vi "QueryLimitTripOffLCDC501.vi"(8 "error in (no error)":errorcluster, 11 "VISA resource name":refnum<visa-resource-name>) -> (0 "error out":errorcluster, 2 "LASER LIMIT & TRIP-OFF":T1, 3 "VISA resource name out":refnum<visa-resource-name>)   [LabVIEW 2021]
panel:
  # "Laser Trip-off on"
  # "Current Limit"
  # "TEC Off"
  # "Min Temperature"
  # "Max Temperature"
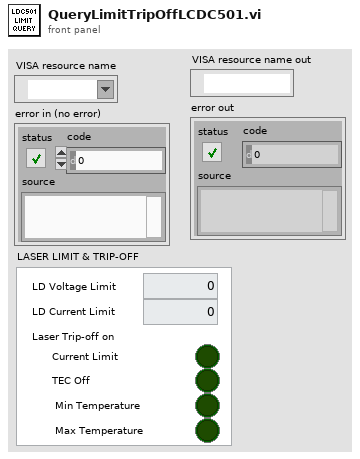
[diagram p1: front panel]
types:
  T1 = cluster{"LD Voltage Limit":dbl, "LD Current Limit":dbl, "Laser Trip-off on Current Limit":bool, "Laser Trip-off on TEC Off":bool, "Laser Trip-off on Min Temperature":bool, "Laser Trip-off on Max Temperature":bool}
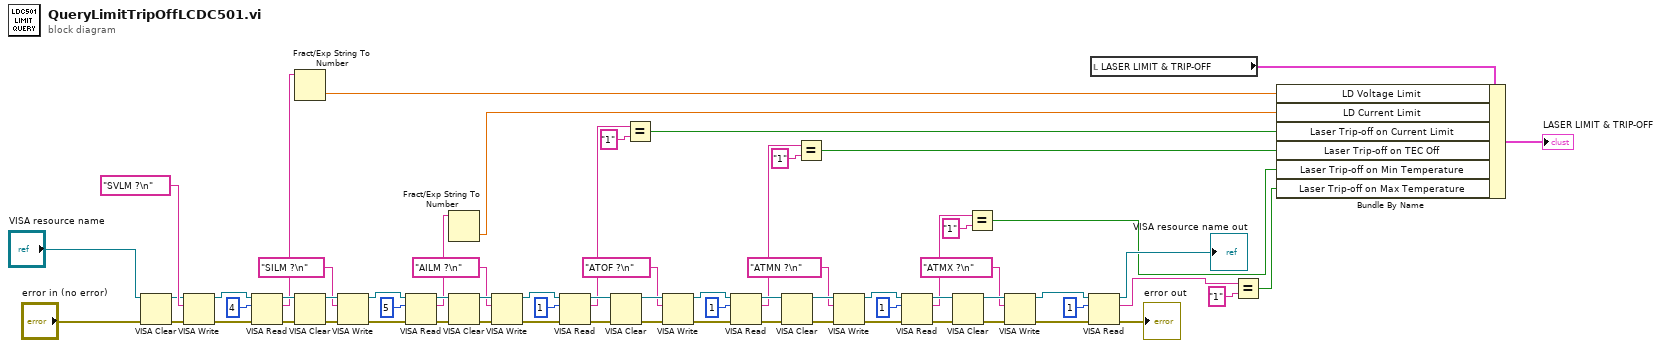
[diagram p0: block diagram]
diagram:
  n1 = VISA Clear(VISA resource name="VISA resource name", error in (no error)="error in (no error)") -> (VISA resource name out=w63:refnum<visa-resource-name>, error out=w64:errorcluster)
  n2 = VISA Write(VISA resource name=w63, write buffer="SVLM ?\n", error in (no error)=w64) -> (VISA resource name out=w67:refnum<visa-resource-name>, error out=w66:errorcluster)  [unwired: 1 out]
  n3 = VISA Read(VISA resource name=w67, byte count=u32 4, error in (no error)=w66) -> (VISA resource name out=w40:refnum<visa-resource-name>, read buffer=w18:string, error out=w39:errorcluster)  [unwired: 1 out]
  n4 = Fract/Exp String To Number(string=w18) -> (number=w8:dbl)  [unwired: 3 in, 1 out]
  n5 = VISA Clear(VISA resource name=w40, error in (no error)=w39) -> (VISA resource name out=w59:refnum<visa-resource-name>, error out=w60:errorcluster)
  n6 = VISA Write(VISA resource name=w59, write buffer="SILM ?\n", error in (no error)=w60) -> (VISA resource name out=w62:refnum<visa-resource-name>, error out=w61:errorcluster)  [unwired: 1 out]
  n7 = VISA Read(VISA resource name=w62, byte count=u32 5, error in (no error)=w61) -> (VISA resource name out=w55:refnum<visa-resource-name>, read buffer=w17:string, error out=w53:errorcluster)  [unwired: 1 out]
  n8 = Fract/Exp String To Number(string=w17) -> (number=w6:dbl)  [unwired: 3 in, 1 out]
  n9 = VISA Clear(VISA resource name=w55, error in (no error)=w53) -> (VISA resource name out=w54:refnum<visa-resource-name>, error out=w56:errorcluster)
  n10 = VISA Write(VISA resource name=w54, write buffer="AILM ?\n", error in (no error)=w56) -> (VISA resource name out=w57:refnum<visa-resource-name>, error out=w58:errorcluster)  [unwired: 1 out]
  n11 = VISA Read(VISA resource name=w57, byte count=u32 1, error in (no error)=w58) -> (VISA resource name out=w48:refnum<visa-resource-name>, read buffer=w15:string, error out=w47:errorcluster)  [unwired: 1 out]
  n12 = VISA Clear(VISA resource name=w48, error in (no error)=w47) -> (VISA resource name out=w49:refnum<visa-resource-name>, error out=w50:errorcluster)
  n13 = Equal?(x=w15, y="1") -> (x = y?=w5:bool)
  n14 = VISA Write(VISA resource name=w49, write buffer="ATOF ?\n", error in (no error)=w50) -> (VISA resource name out=w51:refnum<visa-resource-name>, error out=w52:errorcluster)  [unwired: 1 out]
  n15 = VISA Read(VISA resource name=w51, byte count=u32 1, error in (no error)=w52) -> (VISA resource name out=w44:refnum<visa-resource-name>, read buffer=w13:string, error out=w41:errorcluster)  [unwired: 1 out]
  n16 = VISA Clear(VISA resource name=w44, error in (no error)=w41) -> (VISA resource name out=w43:refnum<visa-resource-name>, error out=w45:errorcluster)
  n17 = Equal?(x=w13, y="1") -> (x = y?=w4:bool)
  n18 = VISA Write(VISA resource name=w43, write buffer="ATMN ?\n", error in (no error)=w45) -> (VISA resource name out=w42:refnum<visa-resource-name>, error out=w46:errorcluster)  [unwired: 1 out]
  n19 = VISA Read(VISA resource name=w42, byte count=u32 1, error in (no error)=w46) -> (VISA resource name out=w24:refnum<visa-resource-name>, read buffer=w11:string, error out=w23:errorcluster)  [unwired: 1 out]
  n20 = VISA Clear(VISA resource name=w24, error in (no error)=w23) -> (VISA resource name out=w28:refnum<visa-resource-name>, error out=w29:errorcluster)
  n21 = Equal?(x=w11, y="1") -> (x = y?=w3:bool)
  n22 = VISA Write(VISA resource name=w28, write buffer="ATMX ?\n", error in (no error)=w29) -> (VISA resource name out=w27:refnum<visa-resource-name>, error out=w30:errorcluster)  [unwired: 1 out]
  n23 = VISA Read(VISA resource name=w27, byte count=u32 1, error in (no error)=w30) -> (VISA resource name out=→"VISA resource name out":refnum<visa-resource-name>, read buffer=w9:string, error out=→"error out":errorcluster)  [unwired: 1 out]
  n24 = local read "LASER LIMIT & TRIP-OFF"() -> (w7:T1)
  n25 = Equal?(x=w9, y="1") -> (x = y?=w2:bool)
  n26 = Bundle By Name(cluster=w7, "LD Voltage Limit"=w8, "LD Current Limit"=w6, "Laser Trip-off on Current Limit"=w5, "Laser Trip-off on TEC Off"=w4, "Laser Trip-off on Min Temperature"=w3, "Laser Trip-off on Max Temperature"=w2) -> (→"LASER LIMIT & TRIP-OFF":T1)
